vi "Adv占空比测量.vi"(0 "通道":enum16{"T1", "T2", "P", "S"}(ring), 3 "error in (no error)":errorcluster) -> (4 "占空比1":dbl[](array[numeric]) format="%.2f", 5 "占空比2":dbl[](array[numeric]) format="%.2f", 7 "占空比1":dbl, 8 "占空比2":dbl, 10 "error out":errorcluster)   [LabVIEW 2020]
uses:
  ed5d0faa-5526-4a4f-8934-9ce51a87c90c.vi
  9380b702-5c5d-44b3-91b2-4898fe6c4266.vi
  <userlib>/_MGI/1D Array/MGI Average/MGI Average (DBL[]).vi
  <userlib>/DAQNavi Polymorphic VI/read/DAQNavi Read (Counter Pulse Width 1Chan 1Samp).vi
  <userlib>/DAQNavi Polymorphic VI/create/DAQNavi Create Channel(CI-PulseWidth).vi
  2500aa03-8c62-4b08-b1ff-c6081716f4ef.vi
  a13042c5-0bc5-48cd-8df0-39ea11c5e7ae.vi
panel:
  in  "error in (no error) 2":errorcluster
  out "error out 2":errorcluster
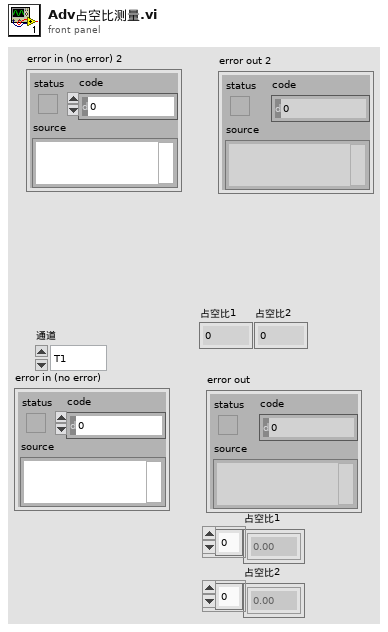
[diagram p1: front panel]
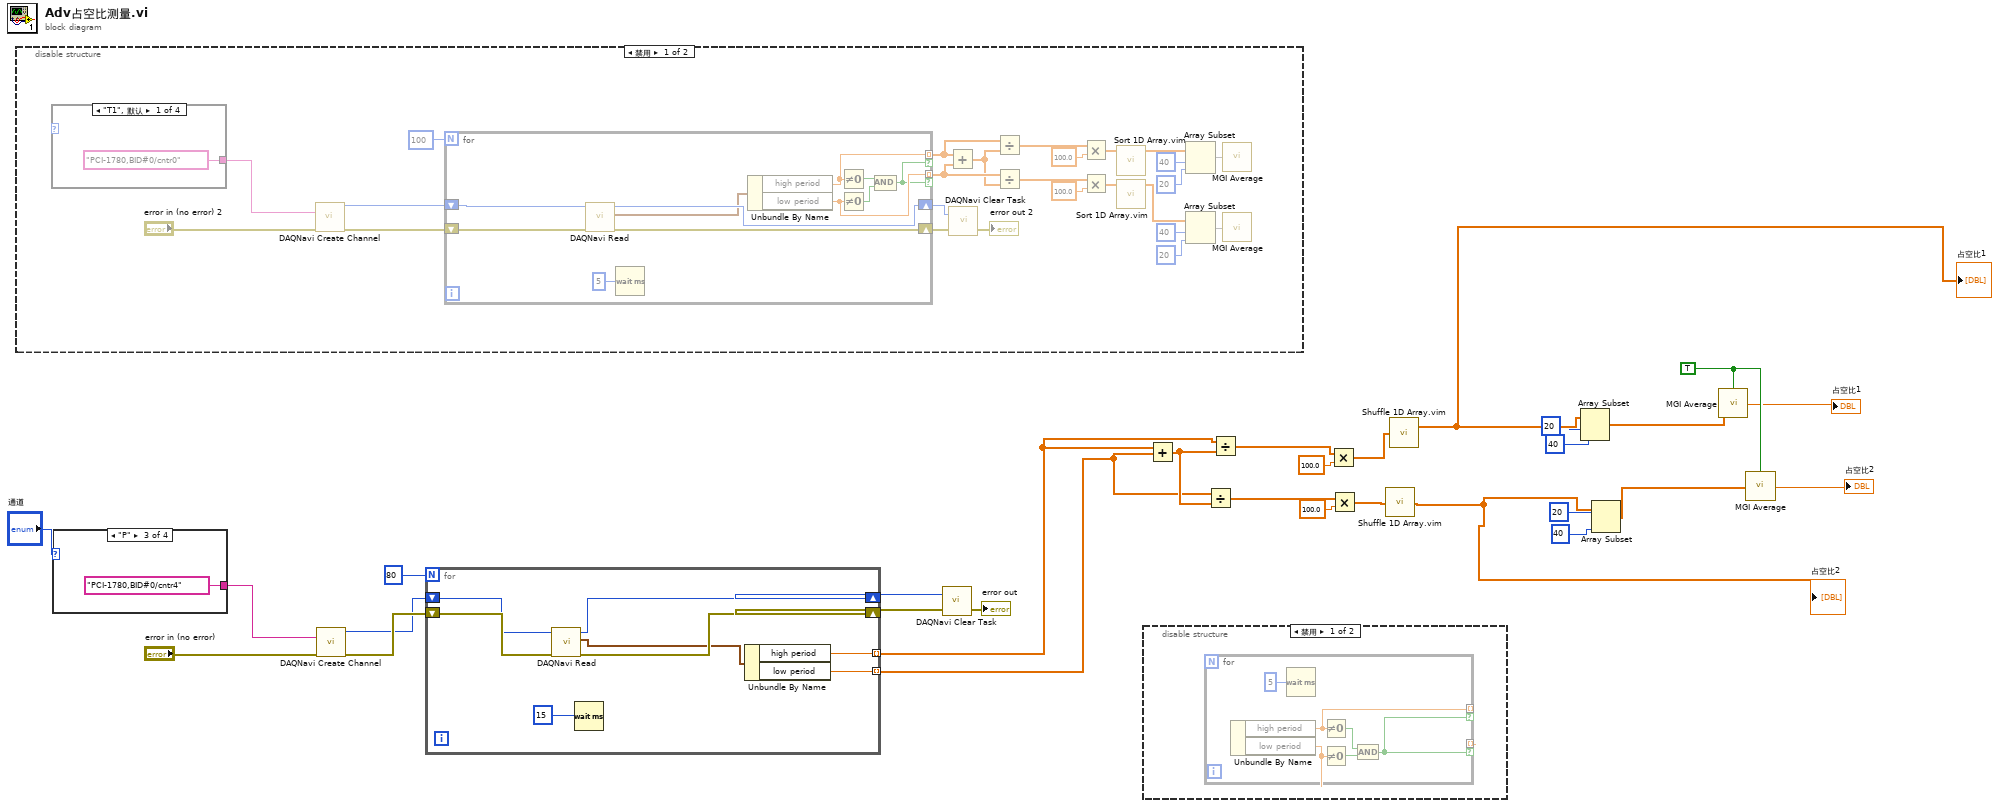
[diagram p0: block diagram]
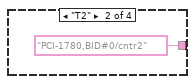
[diagram p3: hidden frame]
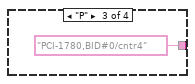
[diagram p4: hidden frame]
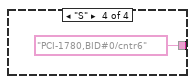
[diagram p5: hidden frame]
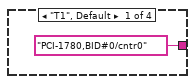
[diagram p7: hidden frame]
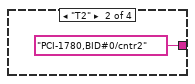
[diagram p8: hidden frame]
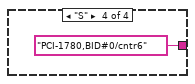
[diagram p9: hidden frame]
diagram:
  w16 = TRUE ("Ignore NaN? (F)")
  n1 = disable-structure shown="禁用" {
    frame Disabled {
      n2 = case shown="\"T1\", 默认" {
        selector: _ -> [_ _ _ _]
        tunnel: ["PCI-1780,BID#0/cntr0" ("physical channels") "PCI-1780,BID#0/cntr2" ("physical channels") "PCI-1780,BID#0/cntr4" ("physical channels") "PCI-1780,BID#0/cntr6" ("physical channels")] -> w30
        frame "T1", Default {
        }
        frame "T2" {
        }
        frame "P" {
        }
        frame "S" {
        }
      }
      n3 = call-poly <userlib>:"DAQNavi Create Channel.vi"("physical channels"=w30, "error in (no error)"="error in (no error) 2") -> ("task out"=w34:i32, "error out"=w31:errorcluster)  [unwired: 12 in]
      n4 = for {
        N: 100 -> [_]
        shift-right: [w64] -> w32
        shift-left: w31 -> [w65]
        shift-right: [w63] -> w33
        shift-left: w34 -> [w62]
        tunnel: [w57] -> w45 mode=indexing if=w55
        tunnel: [w56] -> w46 mode=indexing if=w55
        n5 = call-poly <userlib>:"DAQNavi Read.vi"("error in (no error)"=w65, "task in"=w62) -> ("error out"=w64:errorcluster, "data"=w58:cluster{"high period":dbl, "low period":dbl}, "task out"=w63:i32)  [unwired: 7 in]
        n6 = Wait (ms)(milliseconds to wait=u32 5 ("等待时间（毫秒）")) -> ()  [unwired: 1 out]
        n7 = Unbundle By Name(w58) -> ("high period"=w57:dbl, "low period"=w56:dbl)
        n8 = Not Equal To 0?(x=w57) -> (x != 0?=w59:bool)
        n9 = Not Equal To 0?(x=w56) -> (x != 0?=w60:bool)
        n10 = Compound Arithmetic op=AND ("复合运算")(w59, w60) -> (w55:bool)
      }
      n11 = Add(x=w45, y=w46) -> (x+y=w35:dbl[])
      n12 = call <userlib>:"DAQNavi Clear Task.vi"("error in (no error)"=w32, "task in"=w33) -> ("error out"=→"error out 2":errorcluster)  [unwired: 1 in]
      n13 = Divide(x=w45, y=w35) -> (x/y=w36:dbl[])
      n14 = Divide(x=w46, y=w35) -> (x/y=w37:dbl[])
      n15 = Multiply(x=w36, y=100.0) -> (x*y=w40:dbl[])
      n16 = Multiply(x=w37, y=100.0) -> (x*y=w42:dbl[])
      n17 = call "Sort 1D Array.vim"("unsorted array"=w40) -> ("sorted array"=w47:dbl[])  [unwired: 10 in]
      n18 = call "Sort 1D Array.vim"("unsorted array"=w42) -> ("sorted array"=w51:dbl[])  [unwired: 10 in]
      n19 = Array Subset(array=w47, index=40 ("索引"), length=20 ("长度")) -> (w48:dbl[])
      n20 = Array Subset(array=w51, index=40 ("索引"), length=20 ("长度")) -> (w52:dbl[])
      n21 = call-poly <userlib>:"MGI Average.vi"("Double[]"=w48) -> ()  [unwired: 1 in, 1 out]
      n22 = call-poly <userlib>:"MGI Average.vi"("Double[]"=w52) -> ()  [unwired: 1 in, 1 out]
    }
    frame Enabled {
    }
  }
  n23 = case shown="\"P\"" "通道" {
    tunnel: ["PCI-1780,BID#0/cntr0" ("physical channels") "PCI-1780,BID#0/cntr2" ("physical channels") "PCI-1780,BID#0/cntr4" ("physical channels") "PCI-1780,BID#0/cntr6" ("physical channels")] -> w29
    frame "T1", Default {
    }
    frame "T2" {
    }
    frame "P" {
    }
    frame "S" {
    }
  }
  n24 = call-poly <userlib>:"DAQNavi Create Channel.vi"("physical channels"=w29, "error in (no error)"="error in (no error)") -> ("task out"=w20:i32, "error out"=w21:errorcluster)  [unwired: 12 in]
  n25 = for {
    N: 80 -> [_]
    shift-right: [w79] -> w19
    shift-left: w21 -> [w81]
    shift-right: [w78] -> w18
    shift-left: w20 -> [w80]
    tunnel: [w77] -> w13 mode=indexing
    tunnel: [w76] -> w12 mode=indexing
    n26 = call-poly <userlib>:"DAQNavi Read.vi"("error in (no error)"=w81, "task in"=w80) -> ("error out"=w79:errorcluster, "data"=w75:cluster{"high period":dbl, "low period":dbl}, "task out"=w78:i32)  [unwired: 7 in]
    n27 = Wait (ms)(milliseconds to wait=u32 15 ("等待时间（毫秒）")) -> ()  [unwired: 1 out]
    n28 = Unbundle By Name(w75) -> ("high period"=w77:dbl, "low period"=w76:dbl)
  }
  n29 = call <userlib>:"DAQNavi Clear Task.vi"("error in (no error)"=w19, "task in"=w18) -> ("error out"=→"error out":errorcluster)  [unwired: 1 in]
  n30 = disable-structure shown="禁用" {
    frame Disabled {
      n31 = for {
        tunnel: [w82] -> _ mode=indexing if=w85
        tunnel: [w83] -> _ mode=indexing if=w85
        n32 = Unbundle By Name() -> ("high period"=w83:dbl, "low period"=w82:dbl)  [unwired: 1 in]
        n33 = Wait (ms)(milliseconds to wait=u32 5 ("等待时间（毫秒）")) -> ()  [unwired: 1 out]
        n34 = Not Equal To 0?(x=w83) -> (x != 0?=w86:bool)
        n35 = Not Equal To 0?(x=w82) -> (x != 0?=w87:bool)
        n36 = Compound Arithmetic op=AND ("复合运算")(w86, w87) -> (w85:bool)
      }
    }
    frame Enabled {
    }
  }
  n37 = Add(x=w13, y=w12) -> (x+y=w22:dbl[])
  n38 = Divide(x=w12, y=w22) -> (x/y=w25:dbl[])
  n39 = Divide(x=w13, y=w22) -> (x/y=w26:dbl[])
  n40 = Multiply(x=w26, y=100.0) -> (x*y=w8:dbl[])
  n41 = Multiply(x=w25, y=100.0) -> (x*y=w6:dbl[])
  n42 = call "Shuffle 1D Array.vim"("array"=w6) -> ("shuffled array"=w5:dbl[])  [unwired: 4 in]
  "占空比2" <- w5
  n43 = call "Shuffle 1D Array.vim"("array"=w8) -> ("shuffled array"=w7:dbl[])  [unwired: 4 in]
  "占空比1" <- w7
  n44 = Array Subset(array=w7, index=20 ("索引"), length=40 ("长度")) -> (w11:dbl[])
  n45 = Array Subset(array=w5, index=20 ("索引"), length=40 ("长度")) -> (w10:dbl[])
  n46 = call-poly <userlib>:"MGI Average.vi"("Double[]"=w11, "Ignore NaN? (F)"=w16) -> ("Average"=→"占空比1":dbl)
  n47 = call-poly <userlib>:"MGI Average.vi"("Double[]"=w10, "Ignore NaN? (F)"=w16) -> ("Average"=→"占空比2":dbl)
